vi "Display_data_dates.vi"(1 "String":string) -> (0 "resulting string":string)   [LabVIEW 2020]
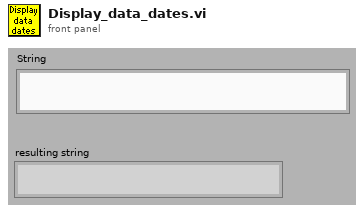
[diagram p1: front panel]
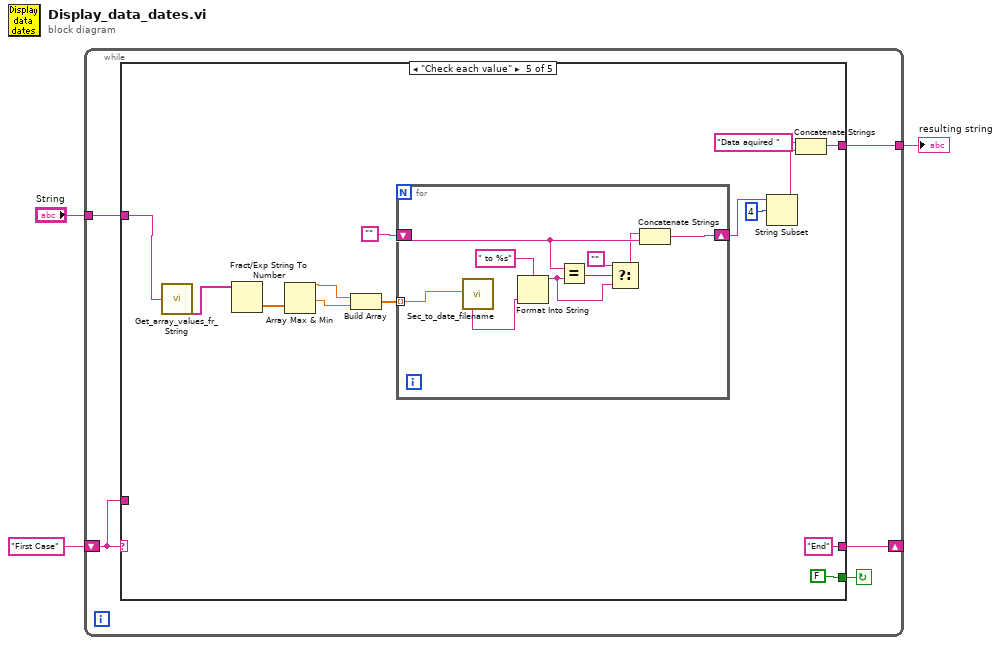
[diagram p0: block diagram]
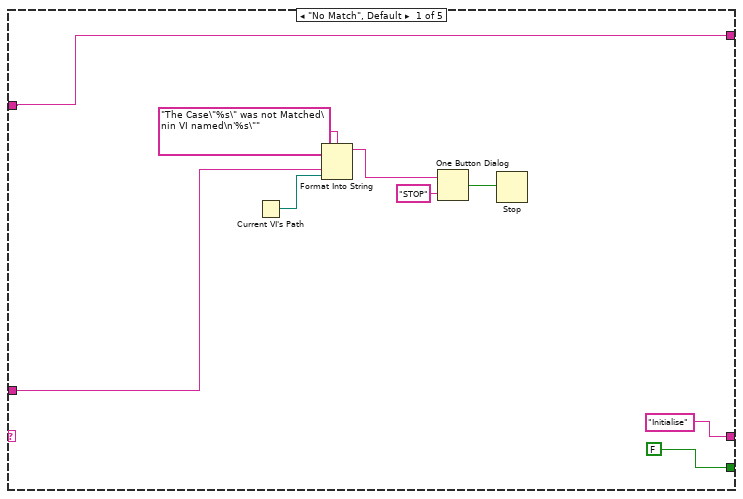
[diagram p2: hidden frame]
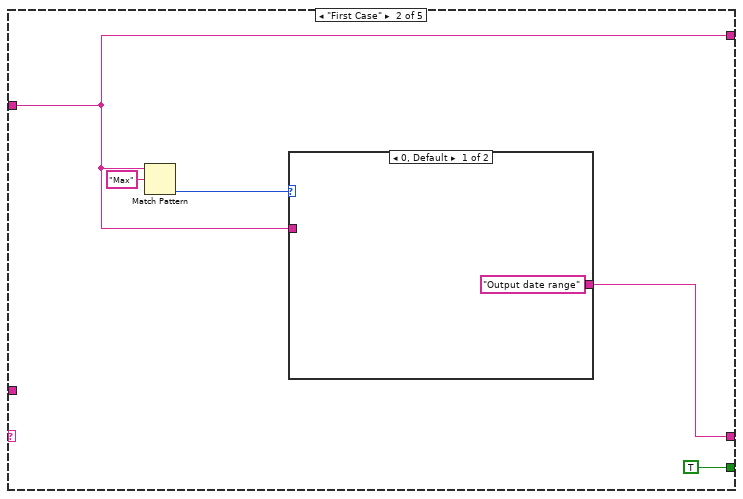
[diagram p3: hidden frame]
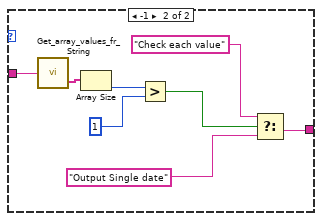
[diagram p4: hidden frame]
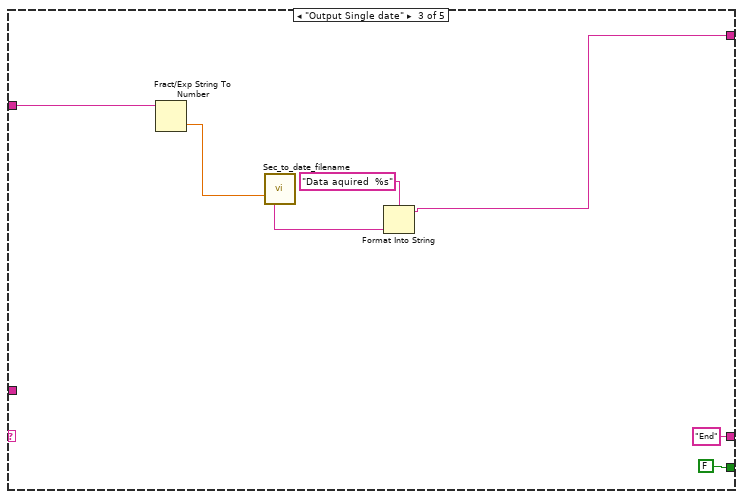
[diagram p5: hidden frame]
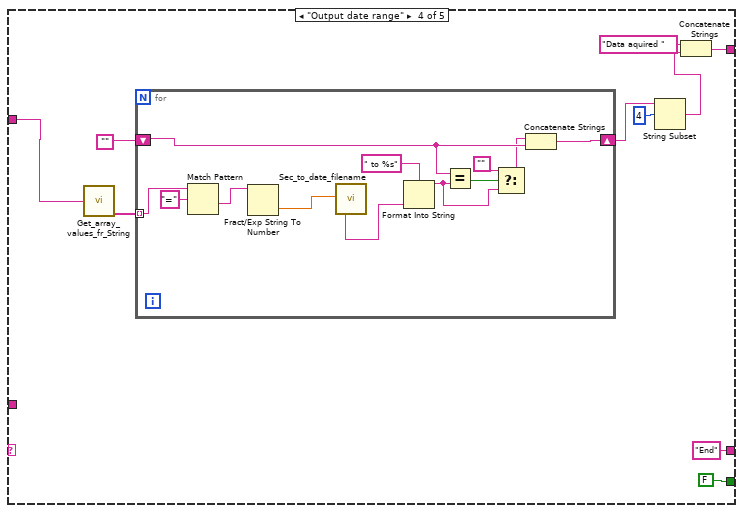
[diagram p6: hidden frame]
diagram:
  n1 = while {
    shift-left: "First Case" -> [w6]
    shift-right: [w7] -> _
    tunnel: "String" -> [w5]
    tunnel: [w4] -> w1
    stop <- w8 continue-if-true
    n2 = case shown="\"Check each value\"" w6 {
      tunnel: [FALSE TRUE FALSE FALSE FALSE] -> w8
      tunnel: ["Initialise" w19 "End" "End" "End"] -> w7
      tunnel: w6 -> [w12 _ _ _ _]
      tunnel: w5 -> [w9 w18 w35 w47 w73]
      tunnel: [w9 w18 w34 w39 w62] -> w4
      frame "No Match", Default {
        n3 = Current VI's Path() -> (path=w11:path)
        n4 = Format Into String(format string="The Case\"%s\" was not Matched\nin VI named\n'%s\"" ("Format String"), w12, w11) -> (resulting string=w15:string)  [unwired: 2 in, 1 out]
        n5 = One Button Dialog(message=w15, button name ("OK")="STOP") -> (true=w13:bool)
        n6 = Stop(stop? (T)=w13) -> ()
      }
      frame "First Case" {
        n7 = Match Pattern(string=w18, regular expression="Max") -> (offset past match=w20:i32)  [unwired: 4 out]
        n8 = case shown="0, Default" w20 {
          tunnel: ["Output date range" w25] -> w19
          tunnel: w18 -> [_ w31]
          frame 0, Default {
          }
          frame -1 {
            n9 = call "Get_array_values_fr_String.vi"("String Value"=w31) -> ("String array"=w30:string[])  [unwired: 1 out]
            n10 = Array Size(array=w30) -> (size(s)=w29:i32)
            n11 = Greater?(x=w29, y=1) -> (0:w27:bool)
            n12 = Select(t="Check each value", s=w27, f="Output Single date") -> (s? t:f=w25:string)
          }
        }
      }
      frame "Output Single date" {
        n13 = Fract/Exp String To Number(string=w35) -> (number=w37:dbl)  [unwired: 4 out]
        n14 = call "Sec_to_date_filename.vi"("ss1904"=w37) -> ("YYYY-mm-DD"=w32:string)  [unwired: 5 in, 9 out]
        n15 = Format Into String(format string="Data aquired  %s", w32) -> (resulting string=w34:string)  [unwired: 2 in, 1 out]
      }
      frame "Output date range" {
        n16 = call "Get_array_values_fr_String.vi"("String Value"=w47) -> ("String array"=w46:string[])  [unwired: 1 out]
        n17 = for {
          tunnel: w46 -> [w59] mode=indexing
          shift-right: [w55] -> w42
          shift-left: "" -> [w54]
          n18 = Match Pattern(string=w59, regular expression="=") -> (after substring=w58:string)  [unwired: 4 out]
          n19 = Fract/Exp String To Number(string=w58) -> (number=w56:dbl)  [unwired: 4 out]
          n20 = call "Sec_to_date_filename.vi"("ss1904"=w56) -> ("YYYY-mm-DD"=w49:string)  [unwired: 5 in, 9 out]
          n21 = Format Into String(format string=" to %s", w49) -> (resulting string=w52:string)  [unwired: 2 in, 1 out]
          n22 = Equal?(x=w54, y=w52) -> (x = y?=w53:bool)
          n23 = Select(t="", s=w53, f=w52) -> (s? t:f=w50:string)
          n24 = Concatenate Strings(w50, w54) -> (w55:string)
        }
        n25 = String Subset(string=w42, offset (0)=4) -> (substring=w40:string)  [unwired: 1 out]
        n26 = Concatenate Strings("Data aquired " ("string"), w40) -> (w39:string)
      }
      frame "Check each value" {
        n27 = call "Get_array_values_fr_String.vi"("String Value"=w73) -> ("String array"=w68:string[])  [unwired: 1 out]
        n28 = Fract/Exp String To Number(string=w68) -> (number=w67:dbl[])  [unwired: 4 out]
        n29 = Array Max & Min(array=w67) -> (max value=w66:dbl, min value=w65:dbl)  [unwired: 2 out]
        n30 = Build Array(w66, w65) -> (w64:dbl[])
        n31 = for {
          shift-right: [w82] -> w69
          shift-left: "" -> [w81]
          tunnel: w64 -> [w76] mode=indexing
          n32 = call "Sec_to_date_filename.vi"("ss1904"=w76) -> ("YYYY-mm-DD"=w75:string)  [unwired: 5 in, 9 out]
          n33 = Format Into String(format string=" to %s", w75) -> (resulting string=w79:string)  [unwired: 2 in, 1 out]
          n34 = Equal?(x=w81, y=w79) -> (x = y?=w80:bool)
          n35 = Select(t="", s=w80, f=w79) -> (s? t:f=w77:string)
          n36 = Concatenate Strings(w77, w81) -> (w82:string)
        }
        n37 = String Subset(string=w69, offset (0)=4) -> (substring=w63:string)  [unwired: 1 out]
        n38 = Concatenate Strings("Data aquired " ("string"), w63) -> (w62:string)
      }
    }
  }
  "resulting string" <- w1
